vi "OpenErrorlogFileError.vi"(8 "error in (no error)":errorcluster, 10 "error":errorcluster, 11 "TCP_Server in":refnum<class "TCP_Server.lvclass">) -> (0 "error out":errorcluster, 3 "TCP_Server out":refnum<class "TCP_Server.lvclass">)   [LabVIEW 2023, in "TCP_Server.lvlib" / "TCP_Server.lvclass"]
uses:
  TCP_Server.lvclass
  TCP_Server.lvclass/TCP_Server.ctl
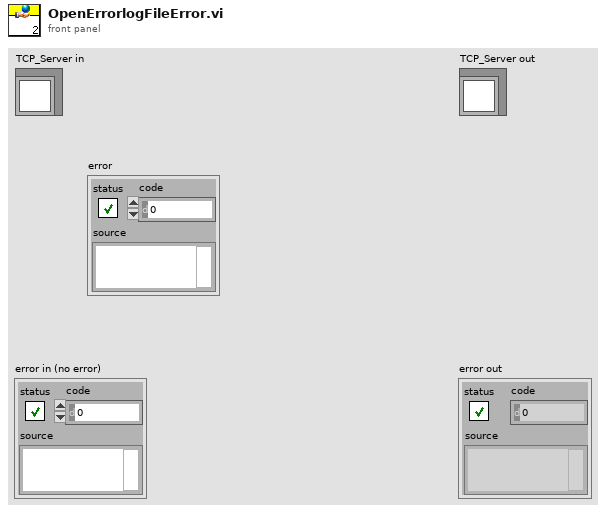
[diagram p1: front panel]
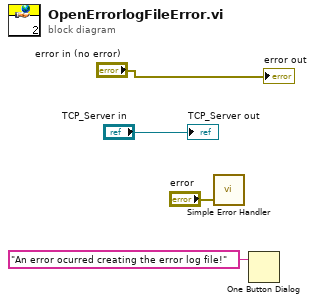
[diagram p0: block diagram]
diagram:
  n1 = call <vilib>:"Simple Error Handler.vi"("error in (no error)"="error") -> ()  [unwired: 4 in, 5 out]
  n2 = One Button Dialog(message="An error ocurred creating the error log file!") -> ()  [unwired: 1 in, 1 out]
  "error out" <- "error in (no error)"
  "TCP_Server out" <- "TCP_Server in"
